vi "Zoom Spectrum.vi"(8 "error in (no error)":errorcluster, 9 "Width (kHz)":dbl=4.0, 10 "f0":dbl, 11 "DP window":refnum<vi>) -> (0 "error out":errorcluster)   [LabVIEW 2015]
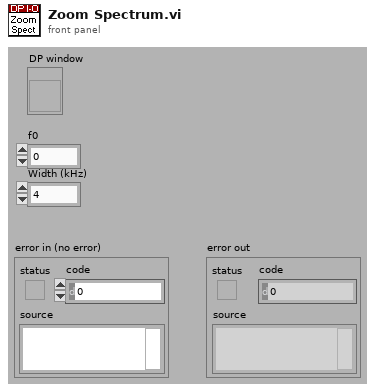
[diagram p1: front panel]
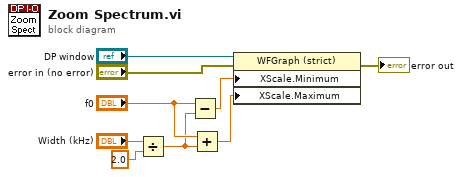
[diagram p0: block diagram]
diagram:
  n1 = Divide(x="Width (kHz)", y=2.0) -> (x/y=w3:dbl)
  n2 = Subtract(x="f0", y=w3) -> (x-y=w2:dbl)
  n3 = Add(x="f0", y=w3) -> (x+y=w1:dbl)
  n4 = property class="WFGraph (strict)"(reference="DP window", error in="error in (no error)", "XScale.Minimum"=w2, "XScale.Maximum"=w1) -> (error out=→"error out":errorcluster)  [unwired: 1 out]
